vi "TriggererExample.vi"() -> ()   [LabVIEW 2012]
panel:
  in  "Acquire":bool
  in  "stop":bool
  in  "Set Other VI's String":bool
  in  "Input String":string
  in  "Init":bool
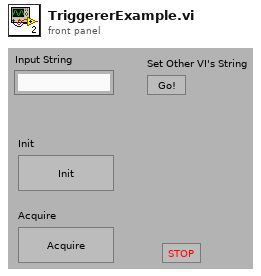
[diagram p1: front panel]
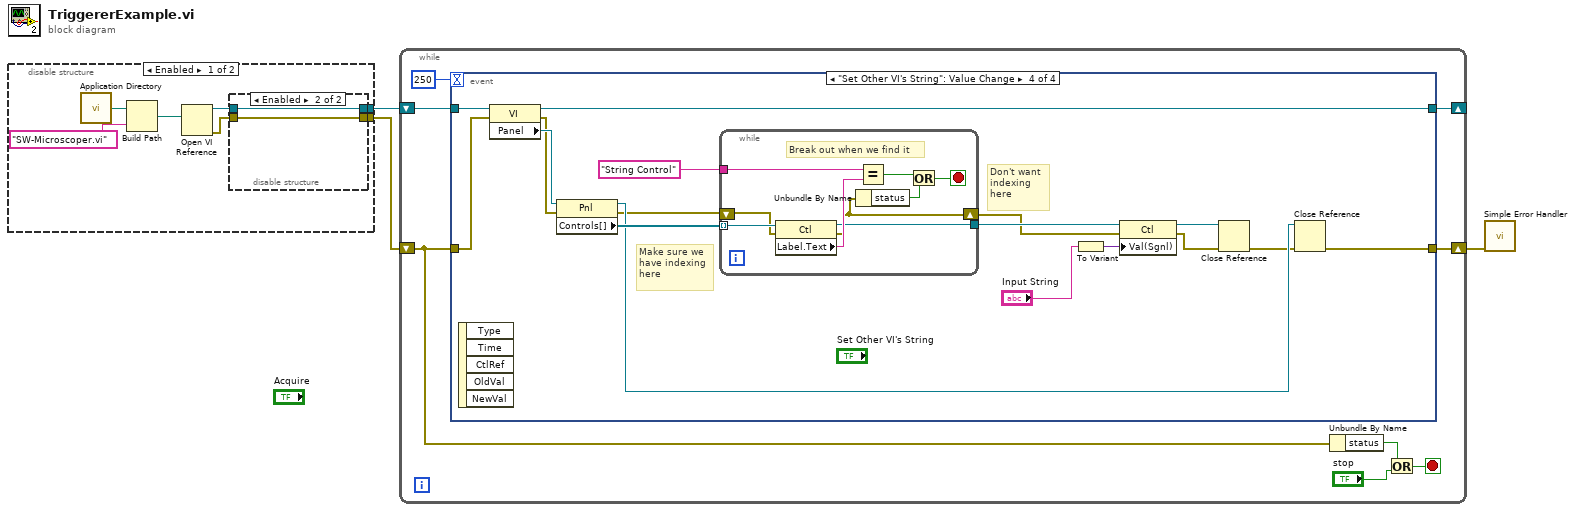
[diagram p0: block diagram]
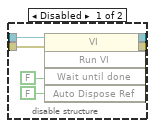
[diagram p2: hidden frame]
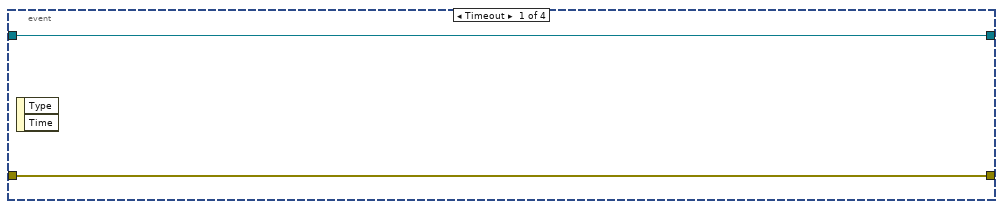
[diagram p4: hidden frame]
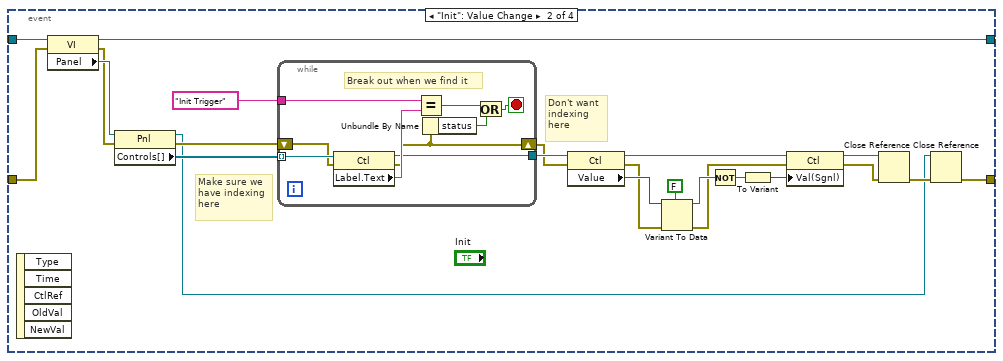
[diagram p5: hidden frame]
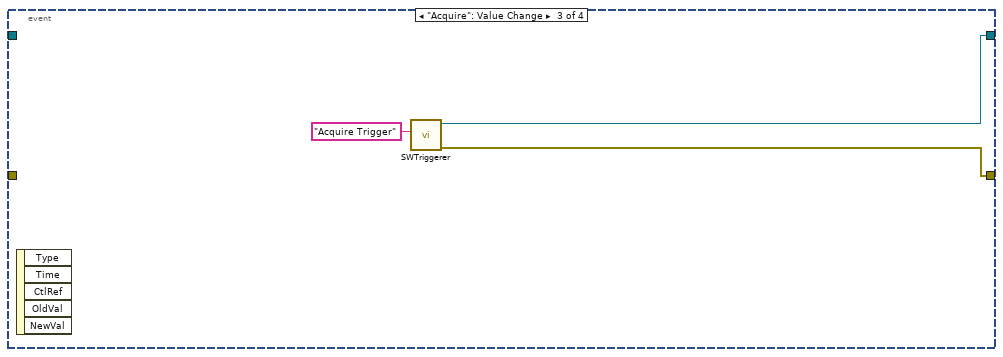
[diagram p6: hidden frame]
diagram:
  n1 = disable-structure shown="Enabled" {
    disable-tunnel: [w5 _] -> w2
    disable-tunnel: [w4 _] -> w1
    frame Enabled {
      n2 = call <vilib>:"Application Directory.vi"() -> ("Application Directory"=w10:path)
      n3 = Build Path(base path=w10, name or relative path="SW-Microscoper.vi") -> (appended path=w8:path)
      n4 = Open VI Reference(vi path=w8) -> (vi reference=w7:refnum<vi>, error out=w6:errorcluster)  [unwired: 5 in]
      n5 = disable-structure shown="Enabled" {
        disable-tunnel: w7 -> [w14 w18]
        disable-tunnel: w6 -> [w13 w17]
        disable-tunnel: [w12 w18] -> w5
        disable-tunnel: [w11 w17] -> w4
        frame Disabled {
          n6 = invoke class="VI" method="Run VI"(reference=w14, error in=w13, "Wait until done"=FALSE ("Front Panel Window:Open"), "Auto Dispose Ref"=FALSE ("Auto Dispose Reference")) -> (reference out=w12:refnum<vi>, error out=w11:errorcluster)  [unwired: 1 in, 3 out]
        }
        frame Enabled {
        }
      }
    }
    frame Disabled {
    }
  }
  n7 = while {
    shift-right: [w26] -> _
    shift-left: w2 -> [w25]
    shift-right: [w24] -> w3
    shift-left: w1 -> [w22]
    stop <- w21 stop-if-true
    n8 = event shown="[3] \"Set Other VI's String\": Value Change" {
      selector: _ -> [_ _ _ _]
      dyn-events: _ -> [_ _ _ _]
      timeout: 250 ("Numeric") -> [_ _ _ _]
      tunnel: w25 -> [w28 w48 _ w77]
      tunnel: [w28 w38 w63 w75] -> w26
      tunnel: [w27 w32 w62 w68] -> w24
      tunnel: w22 -> [w27 w37 _ w67]
      event Timeout {
        n9 = event-data() -> ()  [unwired: 1 in, 2 out]
      }
      event "Init": Value Change {
        # "Don't want\nindexing\nhere"
        # "Make sure we\nhave indexing\nhere"
        n10 = event-data() -> ()  [unwired: 1 in, 5 out]
        n11 = property class="VI"(reference=w48, error in=w37) -> (reference out=w38:refnum<vi>, error out=w36:errorcluster, "Panel"=w51:refnum<vi>)
        n12 = property class="Pnl"(reference=w51, error in=w36) -> (reference out=w29:refnum<vi>, error out=w35:errorcluster, "Controls[]"=w50:refnum<vi>[])
        n13 = while {
          tunnel: w50 -> [w60] mode=indexing
          tunnel: "Init Trigger" ("Control Name") -> [w59]
          tunnel: [w57] -> w47
          shift-right: [w55] -> w34
          shift-left: w35 -> [w56]
          stop <- w54 stop-if-true
          # "Break out when we find it"
          n14 = property class="Ctl"(reference=w60, error in=w56) -> (reference out=w57:refnum<vi>, error out=w55:errorcluster, "Label.Text"=w58:string)
          n15 = Equal?(x=w59, y=w58) -> (x = y?=w52:bool)
          n16 = Unbundle By Name(w55) -> ("status"=w53:bool)
          n17 = Or(x=w52, y=w53) -> (x .or. y?=w54:bool)
        }
        n18 = property class="Ctl"(reference=w47, error in=w34) -> (reference out=w46:refnum<vi>, error out=w40:errorcluster, "Value"=w44:variant)
        n19 = Variant To Data(error in=w40, type=FALSE ("Push Other VI's Button 2"), Variant=w44) -> (data=w41:bool, error out=w39:errorcluster)
        n20 = Not(x=w41) -> (.not. x?=w42:bool)
        n21 = To Variant(anything=w42) -> (Variant=w45:variant)
        n22 = property class="Ctl"(reference=w46, error in=w39, "Val(Sgnl)"=w45) -> (reference out=w30:refnum<vi>, error out=w31:errorcluster)
        n23 = Close Reference(reference=w30, error in (no error)=w31) -> (error out=w33:errorcluster)
        n24 = Close Reference(reference=w29, error in (no error)=w33) -> (error out=w32:errorcluster)
      }
      event "Acquire": Value Change {
        n25 = event-data() -> ()  [unwired: 1 in, 5 out]
        n26 = call "SWTriggerer.vi"("Control Name"="Acquire Trigger") -> ("error out"=w62:errorcluster, "VI out"=w63:refnum<vi>)  [unwired: 9 in]
      }
      event "Set Other VI's String": Value Change {
        # "Don't want\nindexing\nhere"
        # "Make sure we\nhave indexing\nhere"
        n27 = event-data() -> ()  [unwired: 1 in, 5 out]
        n28 = property class="VI"(reference=w77, error in=w67) -> (reference out=w75:refnum<vi>, error out=w66:errorcluster, "Panel"=w80:refnum<vi>)
        n29 = property class="Pnl"(reference=w80, error in=w66) -> (reference out=w71:refnum<vi>, error out=w65:errorcluster, "Controls[]"=w79:refnum<vi>[])
        n30 = while {
          tunnel: w79 -> [w89] mode=indexing
          tunnel: "String Control" ("Control Name") -> [w88]
          tunnel: [w86] -> w73
          shift-right: [w81] -> w64
          shift-left: w65 -> [w85]
          stop <- w82 stop-if-true
          # "Break out when we find it"
          n31 = property class="Ctl"(reference=w89, error in=w85) -> (reference out=w86:refnum<vi>, error out=w81:errorcluster, "Label.Text"=w87:string)
          n32 = Unbundle By Name(w81) -> ("status"=w84:bool)
          n33 = Equal?(x=w88, y=w87) -> (x = y?=w83:bool)
          n34 = Or(x=w83, y=w84) -> (x .or. y?=w82:bool)
        }
        n35 = To Variant(anything="Input String") -> (Variant=w76:variant)
        n36 = property class="Ctl"(reference=w73, error in=w64, "Val(Sgnl)"=w76) -> (reference out=w72:refnum<vi>, error out=w70:errorcluster)
        n37 = Close Reference(reference=w72, error in (no error)=w70) -> (error out=w69:errorcluster)
        n38 = Close Reference(reference=w71, error in (no error)=w69) -> (error out=w68:errorcluster)
      }
    }
    n39 = Unbundle By Name(w22) -> ("status"=w20:bool)
    n40 = Or(x=w20, y="stop") -> (x .or. y?=w21:bool)
  }
  n41 = call <vilib>:"Simple Error Handler.vi"("error in (no error)"=w3) -> ()  [unwired: 4 in, 5 out]
